vi "SPI_TEST.vi"() -> ()   [LabVIEW 2011]
uses:
  <vilib>/rvi/eio/common/nirviEmuTemplateMethod_errors.vi
  <vilib>/eio/EIONode/EIONode.xnode
panel:
  in  "VBatt_ChipSelectInverted":bool
  in  "VBatt_Clock":bool
  out "VBatt_DigitalInput":bool
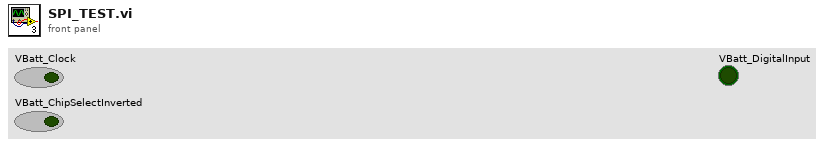
[diagram p1: front panel]
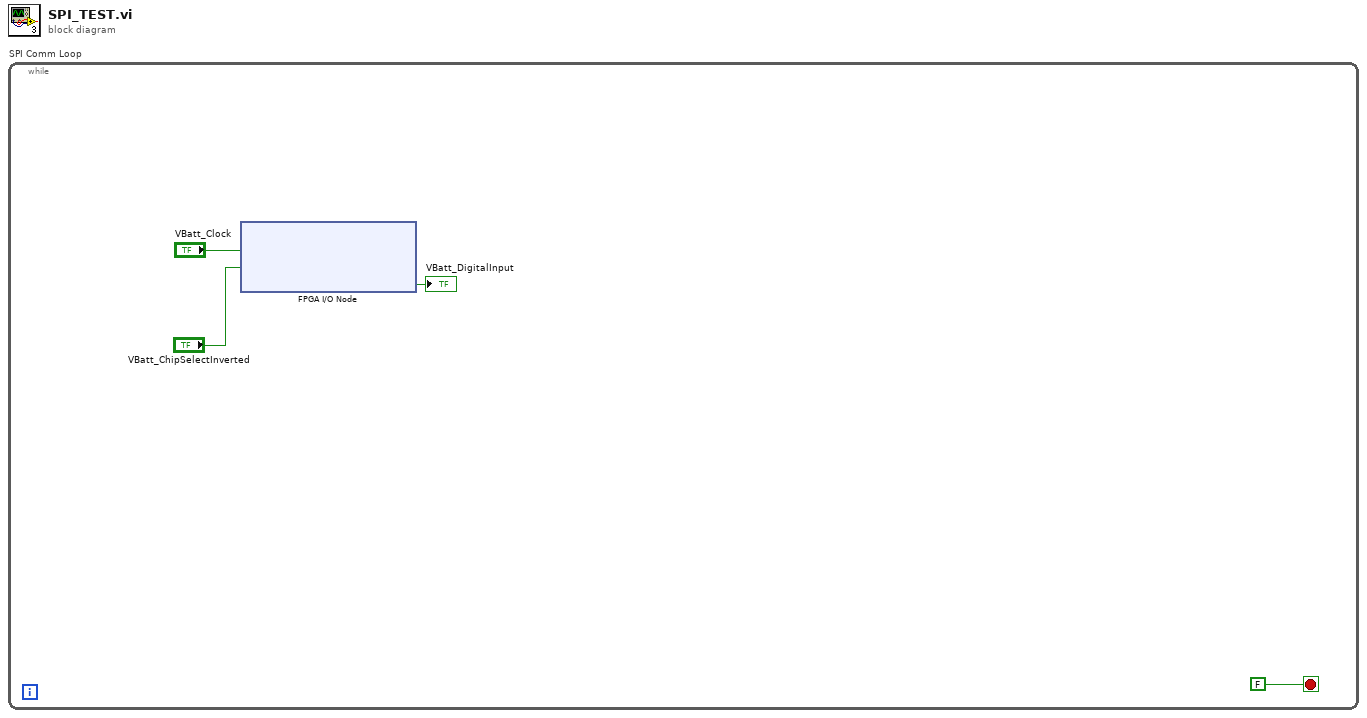
[diagram p0: block diagram]
diagram:
  n1 = while "SPI Comm Loop" {
    stop <- FALSE stop-if-true
    n2 = xnode "FPGA I/O Node"("VBatt_Clock"="VBatt_Clock", "VBatt_ChipSelectInverted"="VBatt_ChipSelectInverted") -> ("VBatt_DigitalInput"=→"VBatt_DigitalInput":bool)  [unwired: 3 in, 3 out]
  }
